vi "Load Hardware.vi"(8 "error in (no error)":errorcluster, 10 "Program only changes":bool=TRUE, 11 "SRS_DS345 in":refnum<class "SRS_DS345.lvclass">) -> (0 "error out":errorcluster, 3 "SRS_DS345 out":refnum<class "SRS_DS345.lvclass">)   [LabVIEW 2013, in "SRS_DS345.lvclass"]
uses:
  SRS_DS345.lvclass
  SRS_DS345.lvclass/SRS_DS345.ctl
  <vilib>/Instr/_visa.llb/VISA Configure Serial Port (Instr).vi
panel:
  # "encapsulate HWI in cluser so each \"last encountered\"\ncan be a different length."
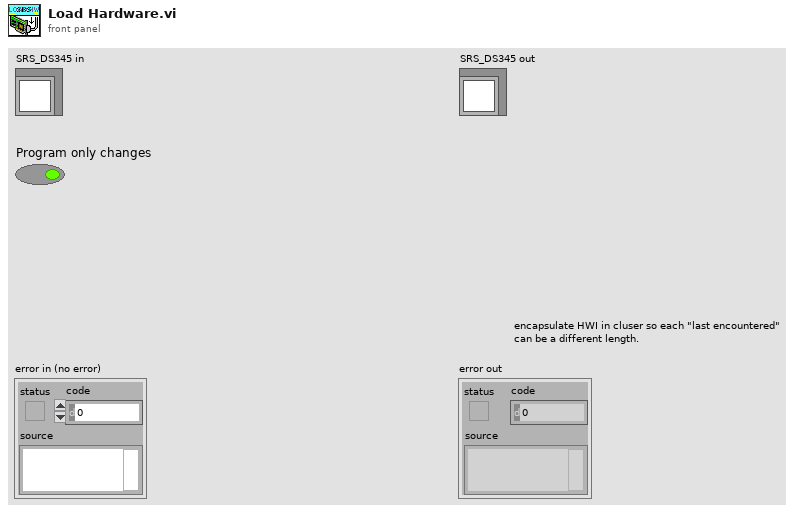
[diagram p1: front panel]
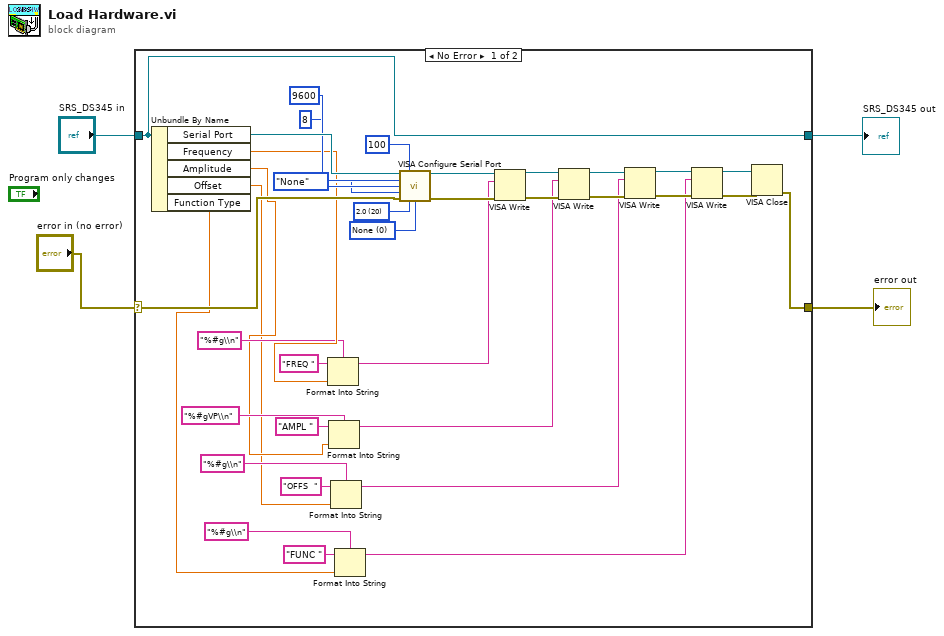
[diagram p0: block diagram]
diagram:
  n1 = case shown="No Error" "error in (no error)" {
    selector: "error in (no error)" -> [w33 w41]
    tunnel: "SRS_DS345 in" -> [w8 w42]
    tunnel: [w8 w42] -> w2
    tunnel: [w5 w41] -> w1
    frame No Error {
      w35 = u16 0 items=["None", "XON/XOFF", "RTS/CTS", "XON/XOFF & RTS/CTS", "DTR/DSR", "XON/XOFF & DTR/DSR"] ("flow control (0:none)")
      w36 = u16 20 items=["1.0"=10, "1.5"=15, "2.0"=20] ("stop bits (10: 1 bit)")
      n2 = Unbundle By Name(w8) -> ("Serial Port"=w40:refnum<visa-resource-name>, "Frequency"=w32:dbl, "Amplitude"=w27:dbl, "Offset"=w22:dbl, "Function Type"=w21:dbl)
      n3 = Format Into String(format string="%#g\\n", initial string="FREQ ", w32) -> (resulting string=w19:string)  [unwired: 1 in, 1 out]
      n4 = Format Into String(format string="%#gVP\\n", initial string="AMPL ", w27) -> (resulting string=w15:string)  [unwired: 1 in, 1 out]
      n5 = Format Into String(format string="%#g\\n", initial string="OFFS  ", w22) -> (resulting string=w10:string)  [unwired: 1 in, 1 out]
      n6 = Format Into String(format string="%#g\\n", initial string="FUNC ", w21) -> (resulting string=w9:string)  [unwired: 1 in, 1 out]
      n7 = call-poly "VISA Configure Serial Port"("VISA resource name"=w40, "timeout (10sec)"=u32 100, "baud rate (9600)"=u32 9600, "data bits (8)"=u16 8, "parity (0:none)"=enum16{"None", "Odd", "Even", "Mark", "Space"}."None", "error in (no error)"=w33, "stop bits (10: 1 bit)"=w36, "flow control (0:none)"=w35) -> ("VISA resource name out"=w18:refnum<visa-resource-name>, "error out"=w20:errorcluster)  [unwired: 6 in]
      n8 = VISA Write(VISA resource name=w18, write buffer=w19, error in (no error)=w20) -> (VISA resource name out=w16:refnum<visa-resource-name>, error out=w17:errorcluster)  [unwired: 1 out]
      n9 = VISA Write(VISA resource name=w16, write buffer=w15, error in (no error)=w17) -> (VISA resource name out=w14:refnum<visa-resource-name>, error out=w12:errorcluster)  [unwired: 1 out]
      n10 = VISA Write(VISA resource name=w14, write buffer=w10, error in (no error)=w12) -> (VISA resource name out=w13:refnum<visa-resource-name>, error out=w11:errorcluster)  [unwired: 1 out]
      n11 = VISA Write(VISA resource name=w13, write buffer=w9, error in (no error)=w11) -> (VISA resource name out=w7:refnum<visa-resource-name>, error out=w6:errorcluster)  [unwired: 1 out]
      n12 = VISA Close(VISA resource name=w7, error in (no error)=w6) -> (error out=w5:errorcluster)
    }
    frame Error {
    }
  }
  "error out" <- w1
  "SRS_DS345 out" <- w2
